vi "SIAM-send.vi"(5 "Value":i32, 7 "connection ID":refnum<k5>, 8 "error in (no error)":errorcluster, 10 "Script":T2(array[cluster])=[{"Delay 10µs"=0, "command"=4027514895, "P0"=5, "P1"=0, "P2"=0, "P3"=0, "P4"=0, "P5-ticket"=0}] {"command" format="%x" items=["read_x-Motor_status_ticket"=17305600, "init_x-Motor"=17760263, "read_x-Motor_absolute_ticket"=16781312, "move_x-Motor_absolute"=16777217, "move_x-Motor_relative"=16842753, "read_y-Motor_status_ticket"=18354176, "init_y-Motor"=18808839, "read_y-Motor_absolute_ticket"=17829888, "move_y-Motor_absolute"=17825793, "move_y-Motor_relative"=17891329, "read_z-Motor_status_ticket"=19402752, "init_z-Motor"=19857415, "stop_z-Motor"=19857423, "start_z-Motor"=19857422, "read_z-Motor_absolute_ticket"=18878464, "move_z-Motor_absolute"=18874369, "move_z-Motor_relative"=18939905, "end_no_ticket"=4027514895, "end_ticket"=4027518991, "IO-read_bank0"=218107904, "IO-write_bank0"=218103809, "IO-read_bank1"=219156480, "IO-write_bank1"=219152385, "IO-delay_bank0"=218365953, "IO-delay_bank0_fromVar"=218365955, "read_cam_clock"=3289124864, "store_cam_clock"=3289120770, "read_cam_phase"=3289190400, "set_cam_deadtime"=3288989697, "set_cam_10uscycles"=3289055233, "set_cam_10uscycles_fromVariable"=3289055235, "calc_cam"=3289317386, "store_cam_Var"=3289251842, "math_addToVariable"=4060086278, "readVar"=4060090368, "writeVar"=4060086273, "copyVar"=4060086276, "decrement_branchRel_if_equal"=4043374945, "decrement_branchRel_if_greaterequal"=4043375201, "decrement_branchRel_if_greaterequal_withTicket"=4043379297, "decrement_branchRel_if_smaller"=4043375457, "increment_branchRel_if_smaller"=4043375473, "writeTMSI"=100663297, "writeTMSI_fromVar"=100663299]}, 11 "command":T3) -> (0 "error out":errorcluster, 2 "Status":enum16{"unknown", "idle", "running", ""}(ring))   [LabVIEW 2011]
uses:
  SIAM-send.ctl
  SIAM_command.ctl
panel:
  # "store locally to allow usage from other vi's"
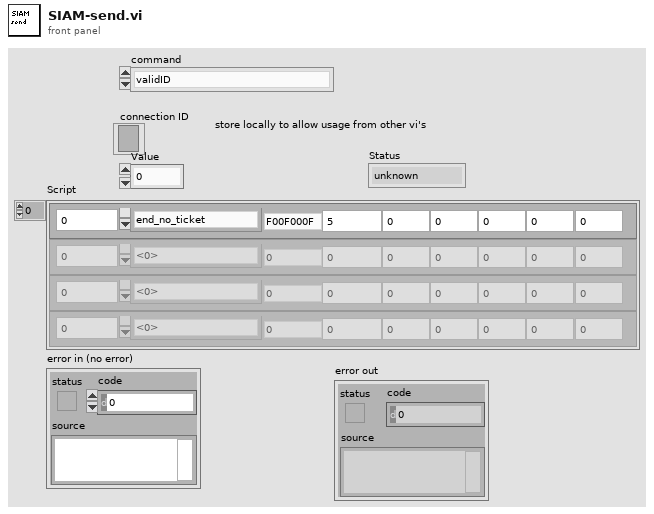
[diagram p1: front panel]
types:
  T1 = typedef "SIAM_command.ctl" = u32
  T2 = cluster{"Delay 10µs":u32, "command":T1, "P0":i32, "P1":i32, "P2":i32, "P3":i32, "P4":i32, "P5-ticket":i32}[]
  T3 = typedef "SIAM-send.ctl" = enum16{"validID", "storeID", "enable", "rundirect", "sendlist", "run", "stop", "readRegister", "sendValue", "storeStatus"}
  T4 = cluster{"Delay 10µs":u32, "command":T1, "P0":i32, "P1":i32, "P2":i32, "P3":i32, "P4":i32, "P5-ticket":i32}
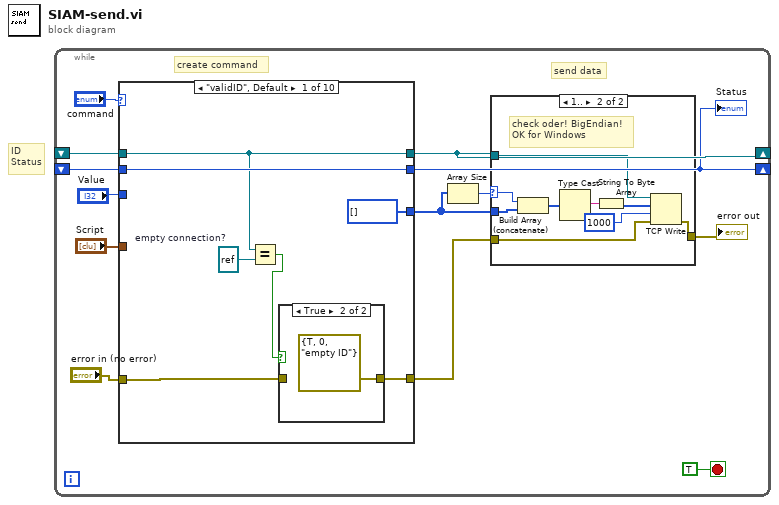
[diagram p0: block diagram]
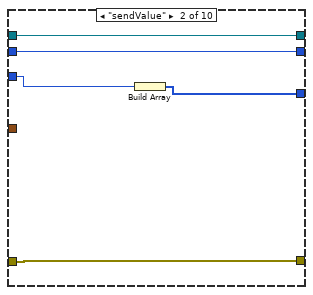
[diagram p4: hidden frame]
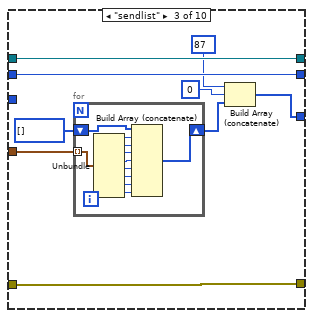
[diagram p5: hidden frame]
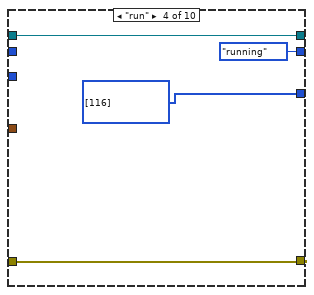
[diagram p6: hidden frame]
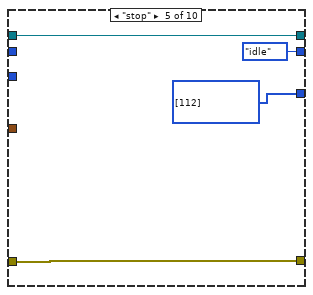
[diagram p7: hidden frame]
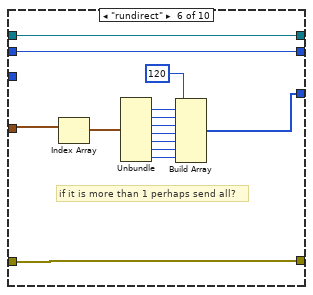
[diagram p8: hidden frame]
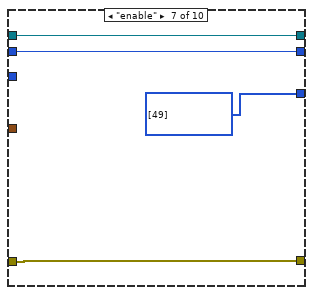
[diagram p9: hidden frame]
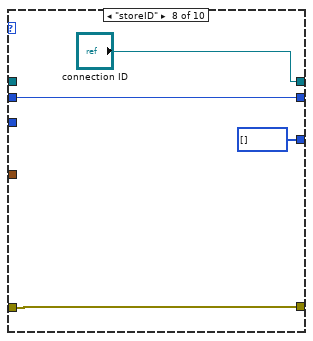
[diagram p10: hidden frame]
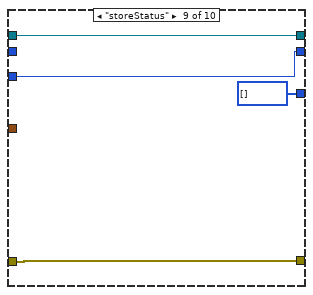
[diagram p11: hidden frame]
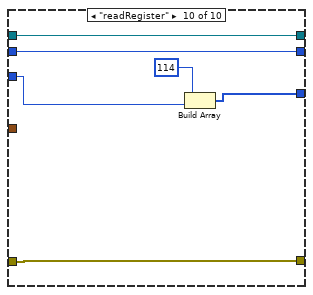
[diagram p12: hidden frame]
diagram:
  # "ID\nStatus"
  n1 = while {
    shift-right: [w5] -> _
    shift-left: _ -> [w11]
    shift-right: [w2] -> _
    shift-left: _ -> [w10]
    stop <- TRUE stop-if-true
    # "send data"
    # "create command"
    n2 = case shown="\"validID\", Default" "command" {
      tunnel: [w28 w36 w46 w61 w64 w78 w83 "connection ID" w91 w97] -> w5
      tunnel: w11 -> [w28 w36 w46 w61 w64 w78 w83 _ w91 w97]
      tunnel: [w30 w37 w45 enum16{"unknown", "idle", "running", ""}."running" ("Status") enum16{"unknown", "idle", "running", ""}."idle" ("Status") w77 w82 w86 w88 w96] -> w2
      tunnel: w10 -> [w30 w37 w45 _ _ w77 w82 w86 _ w96]
      tunnel: "Script" -> [_ _ w43 _ _ w79 _ _ _ _]
      tunnel: "error in (no error)" -> [w25 w35 w44 w60 w62 w76 w80 w84 w89 w94]
      tunnel: [w24 w35 w44 w60 w62 w76 w80 w84 w89 w94] -> w6
      tunnel: [u32[] [] w33 w40 i32[] [116] i32[] [112] w66 i32[] [49] u32[] [] u32[] [] w92] -> w3
      tunnel: "Value" -> [_ w34 _ _ _ _ _ _ w88 w93]
      frame "validID", Default {
        w27 = refnum<k5> refnum  # empty connection?
        n3 = Equal?(x=w28, y=w27) -> (x = y?=w26:bool)
        n4 = case shown="True" w26 {
          tunnel: w25 -> [w31 _]
          tunnel: [w31 errorcluster {"status"=TRUE, "code"=0, "source"="empty ID"} ("error in (no error)")] -> w24
          frame False {
          }
          frame True {
          }
        }
      }
      frame "sendValue" {
        n5 = Build Array(w34) -> (w33:i32[])
      }
      frame "sendlist" {
        n6 = for {
          tunnel: w43 -> [w57] mode=indexing
          shift-right: [w47] -> w41
          shift-left: u32[] [] -> [w48]
          n7 = Unbundle(w57) -> ("Delay 10µs"=w56:u32, "command"=w55:T1, "P0"=w54:i32, "P1"=w53:i32, "P2"=w52:i32, "P3"=w51:i32, "P4"=w50:i32, "P5-ticket"=w49:i32)
          n8 = Build Array (concatenate)(w48, w56, w55, w54, w53, w52, w51, w50, w49) -> (w47:T1[])
        }
        n9 = Build Array (concatenate)(87, u32 0 ("element"), w41) -> (w40:T1[])
      }
      frame "run" {
      }
      frame "stop" {
      }
      frame "rundirect" {
        # "if it is more than 1 perhaps send all?"
        n10 = Index Array(array=w79) -> (element=w75:T4)  [unwired: 1 in]
        n11 = Unbundle(w75) -> ("command"=w74:T1, "P0"=w73:i32, "P1"=w72:i32, "P2"=w71:i32, "P3"=w70:i32, "P4"=w69:i32, "P5-ticket"=w68:i32)  [unwired: 1 out]
        n12 = Build Array(120, w74, w73, w72, w71, w70, w69, w68) -> (w66:T1[])
      }
      frame "enable" {
      }
      frame "storeID" {
      }
      frame "storeStatus" {
      }
      frame "readRegister" {
        n13 = Build Array(114, w93) -> (w92:i32[])
      }
    }
    "Status" <- w2
    n14 = Array Size(array=w3) -> (size(s)=w4:i32)
    n15 = case shown="1.." w4 {
      selector: w4 -> [_ w15]
      tunnel: [w14 w23] -> w7
      tunnel: w6 -> [w14 w22]
      tunnel: w5 -> [_ w21]
      tunnel: w3 -> [_ w16]
      frame 0, Default {
        # "nothing to send"
      }
      frame 1.. {
        # "check oder! BigEndian!\nOK for Windows"
        n16 = Build Array (concatenate)(w15, w16) -> (w19:T1[])
        n17 = Type Cast(x=w19) -> (*(type *) &x=w18:string)  [unwired: 1 out]
        n18 = String To Byte Array(string=w18) -> (unsigned byte array=w17:u8[])
        n19 = TCP Write(connection ID=w21, data in=w17, error in (no error)=w22, 9:1000 ("timeout ms (25000)")) -> (error out=w23:errorcluster)  [unwired: 2 out]
      }
    }
    "error out" <- w7
  }
